vi "Electronic Procedure Debug.vi"() -> ()   [LabVIEW 2017]
panel:
  in  "stop":bool
  in  "CTAH outlet temperature":dbl
  in  "mass flow rate":dbl
  in  "NG flow rate":dbl
  in  "shaft RPM":dbl
  in  "NG pressure in":dbl
  in  "NG temperature in":dbl
  in  "LPT pressure ratio":dbl
  in  "HPT pressure ratio":dbl
  in  "CTAH frequency":dbl
  in  "desired power":dbl
  in  "pump frequency":dbl
  # "Do NOT run this during an experiment!"
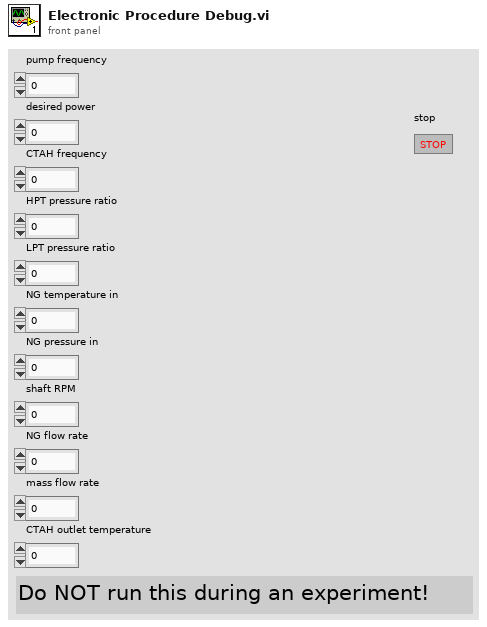
[diagram p1: front panel]
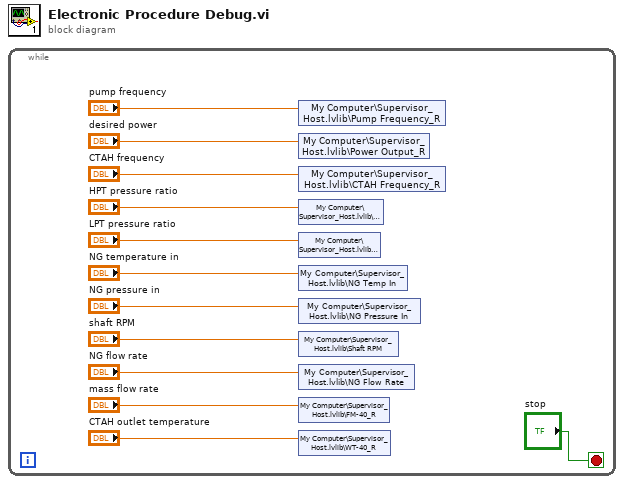
[diagram p0: block diagram]
diagram:
  n1 = while {
    stop <- "stop" stop-if-true
    n2 = shared-variable "My Computer\\Supervisor_Host.lvlib\\Pump Frequency_R"("pump frequency") -> ()  [unwired: 1 in, 1 out]
    n3 = shared-variable "My Computer\\Supervisor_Host.lvlib\\Power Output_R"("desired power") -> ()  [unwired: 1 in, 1 out]
    n4 = shared-variable "My Computer\\Supervisor_Host.lvlib\\CTAH Frequency_R"("CTAH frequency") -> ()  [unwired: 1 in, 1 out]
    n5 = shared-variable "My Computer\\Supervisor_Host.lvlib\\HPT PR"("HPT pressure ratio") -> ()  [unwired: 1 in, 1 out]
    n6 = shared-variable "My Computer\\Supervisor_Host.lvlib\\LPT PR"("LPT pressure ratio") -> ()  [unwired: 1 in, 1 out]
    n7 = shared-variable "My Computer\\Supervisor_Host.lvlib\\NG Temp In"("NG temperature in") -> ()  [unwired: 1 in, 1 out]
    n8 = shared-variable "My Computer\\Supervisor_Host.lvlib\\NG Pressure In"("NG pressure in") -> ()  [unwired: 1 in, 1 out]
    n9 = shared-variable "My Computer\\Supervisor_Host.lvlib\\Shaft RPM"("shaft RPM") -> ()  [unwired: 1 in, 1 out]
    n10 = shared-variable "My Computer\\Supervisor_Host.lvlib\\NG Flow Rate"("NG flow rate") -> ()  [unwired: 1 in, 1 out]
    n11 = shared-variable "My Computer\\Supervisor_Host.lvlib\\FM-40_R"("mass flow rate") -> ()  [unwired: 1 in, 1 out]
    n12 = shared-variable "My Computer\\Supervisor_Host.lvlib\\WT-40_R"("CTAH outlet temperature") -> ()  [unwired: 1 in, 1 out]
  }
